vi "test PantiltMove.vi"(11 "PelcoD frame":string="ÿ\u0002\u0000\u0000\u0000\u0000\u0002") -> (3 "Pantilt Move?":bool)   [LabVIEW 2018]
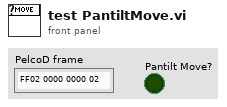
[diagram p1: front panel]
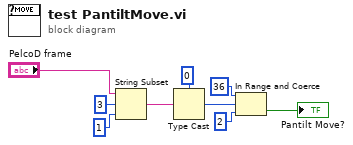
[diagram p0: block diagram]
diagram:
  n1 = String Subset(string="PelcoD frame", offset (0)=3, length (rest)=1 ("length (rest)")) -> (substring=w6:string)
  n2 = Type Cast(type=u8 0, x=w6) -> (*(type *) &x=w4:u8)
  n3 = In Range and Coerce(upper limit=u8 36, x=w4, lower limit=u8 2) -> (In Range?=→"Pantilt Move?":bool)  [unwired: 1 out]
